vi "FPGA_IO.vi"() -> ()   [LabVIEW 2017]
uses:
  <vilib>/rvi/Emulation/niFpgaGetClockAttributes.vi
  <vilib>/rvi/Emulation/niFpgaSctlEmulationGetInTimedLoop.vi
  <vilib>/rvi/Emulation/niFpgaEmulationReportErrorSimple.vi
  <vilib>/rvi/eio/common/nirviEmuTemplateMethod_errors.vi
  <vilib>/rvi/Emulation/niFpgaCriticalErrorInLSC.vi
  <vilib>/eio/EIONode/EIONode.xnode
panel:
  out "output2_read":u16
  out "output1_read":u16
  in  "x3_read":sgl(slide) scale=-10.0..10.0
  in  "x2_read":sgl(slide) scale=-10.0..10.0
  in  "x1_read":sgl(slide) scale=-10.0..10.0
  in  "stop":bool
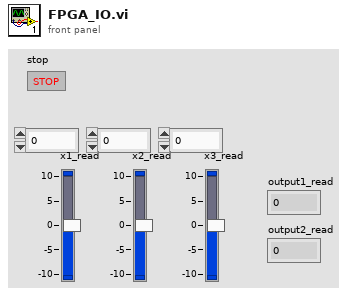
[diagram p1: front panel]
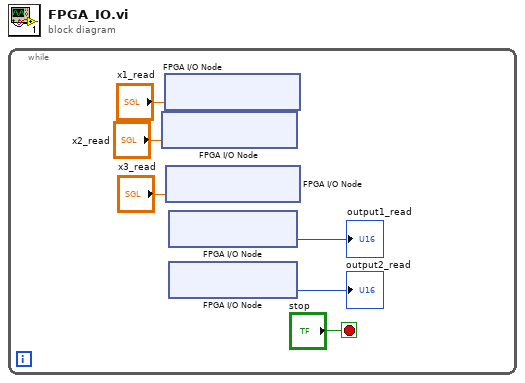
[diagram p0: block diagram]
diagram:
  n1 = while {
    stop <- "stop" stop-if-true
    n2 = xnode "FPGA I/O Node"("ConnectorA/AO1"="x2_read") -> ()  [unwired: 1 in, 1 out]
    n3 = xnode "FPGA I/O Node"("ConnectorA/AO0"="x1_read") -> ()  [unwired: 1 in, 1 out]
    n4 = xnode "FPGA I/O Node"("ConnectorB/AO0"="x3_read") -> ()  [unwired: 1 in, 1 out]
    n5 = xnode "FPGA I/O Node"() -> ("ConnectorB/AI0"=→"output1_read":u16)  [unwired: 1 in, 1 out]
    n6 = xnode "FPGA I/O Node"() -> ("ConnectorB/AI1"=→"output2_read":u16)  [unwired: 1 in, 1 out]
  }
